vi "Set_OI_remote.vi"() -> ()   [LabVIEW 2016]
uses:
  Instrument_Setup.vi
panel:
  out "Address.Communication 3":enum16{"RS232", "ISOBUS", "GPIB", "Gateway"}(ring)
  out "Address.Communication 2":enum16{"RS232", "ISOBUS", "GPIB", "Gateway"}(ring)
  out "Address.Communication":enum16{"RS232", "ISOBUS", "GPIB", "Gateway"}(ring)
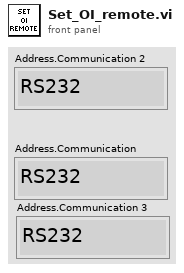
[diagram p1: front panel]
types:
  T1 = typedef "ITCVersion.ctl" = enum16{"ITC502", "ITC503", "ITC601"}
  T2 = cluster{"Version":T1, "ControlTITC":i8, "ControlTCh":i8, "SampleTITC":i8, "SampleTCh":i8, "Instrument address":cluster{"Com Port":i32, "ISOBUS Address":i32, "GPIB Address":i16, "Communication":enum16{"RS232", "ISOBUS", "GPIB", "Gateway"}}}
  T3 = cluster{"Com Port":i32, "ISOBUS Address":i32, "GPIB Address":i16, "Communication":enum16{"RS232", "ISOBUS", "GPIB", "Gateway"}}
  T4 = typedef "PSIO.ctl" = cluster{"Address":T5, "Version":enum16{"PS", "IPS"}}
  T5 = typedef "OxfordAddress.ctl" = cluster{"Com Port":i32, "ISOBUS Address":i32, "GPIB Address":i16, "Communication":enum16{"RS232", "ISOBUS", "GPIB", "Gateway"}}
  T6 = cluster{"Version\n":string, "Max Sweep(4.2K)":dbl[unit], "Max Sweep(2.2K)":dbl[unit], "Switch htr dly":dbl[unit], "Max Field(4.2K)":dbl[unit], "Max Field(2.2K)":dbl[unit], "Max lead res":dbl[unit], "IO Info":T4}
  T7 = cluster{"Display Channel":i32[], "Instrument address":cluster{"Com Port":i32, "ISOBUS Address":i32, "GPIB Address":i16, "Communication":enum16{"RS232", "ISOBUS", "GPIB", "Gateway"}}}
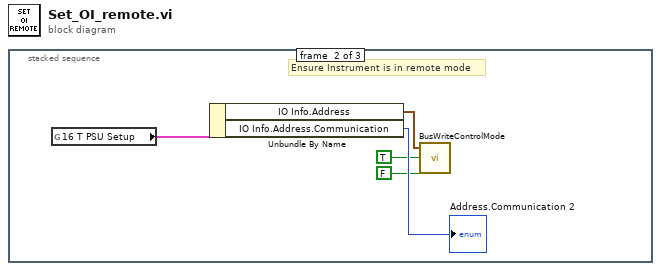
[diagram p0: block diagram]
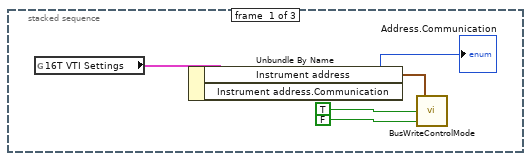
[diagram p2: hidden frame]
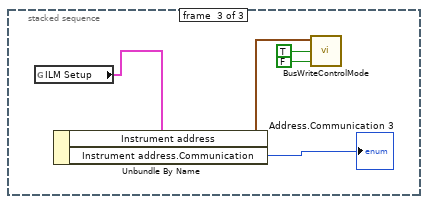
[diagram p3: hidden frame]
diagram:
  n1 = stacked-sequence {
    frame #0 {
      n2 = global read "Instrument_Setup.vi" "16T VTI Settings"() -> (w2:T2)
      n3 = Unbundle By Name(w2) -> ("Instrument address"=w5:T3, "Instrument address.Communication"=→"Address.Communication":enum16{"RS232", "ISOBUS", "GPIB", "Gateway"})
      n4 = call "BusWriteControlMode.vi"("Locked"=FALSE, "Remote"=TRUE, "Address"=w5) -> ()  [unwired: 1 out]
    }
    frame #1 {
      # "Ensure Instrument is in remote mode"
      n5 = global read "Instrument_Setup.vi" "16 T PSU Setup"() -> (w9:T6)
      n6 = Unbundle By Name(w9) -> ("IO Info.Address"=w8:T5, "IO Info.Address.Communication"=→"Address.Communication 2":enum16{"RS232", "ISOBUS", "GPIB", "Gateway"})
      n7 = call "BusWriteControlMode.vi"("Locked"=FALSE, "Remote"=TRUE, "Address"=w8) -> ()  [unwired: 1 out]
    }
    frame #2 {
      n8 = global read "Instrument_Setup.vi" "ILM Setup"() -> (w14:T7)
      n9 = Unbundle By Name(w14) -> ("Instrument address"=w13:T3, "Instrument address.Communication"=→"Address.Communication 3":enum16{"RS232", "ISOBUS", "GPIB", "Gateway"})
      n10 = call "BusWriteControlMode.vi"("Locked"=FALSE, "Remote"=TRUE, "Address"=w13) -> ()  [unwired: 1 out]
    }
  }
